vi "Read Display Name.vi"(11 "Assert Display in":refnum<class "Assert Display.lvclass">) -> (2 "Display Name":string)   [LabVIEW 2016, in "Assert API Components.lvlib" / "Assert Display.lvlib" / "Assert Display.lvclass"]
uses:
  Assert Display.lvclass
  Assert Display.lvclass/Assert Display.ctl
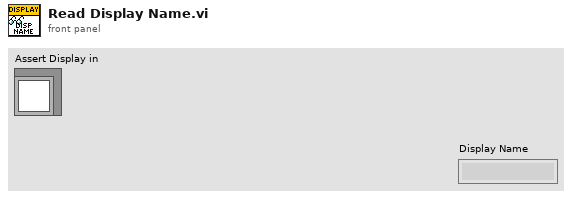
[diagram p1: front panel]
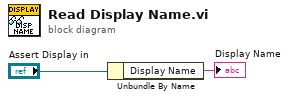
[diagram p0: block diagram]
diagram:
  n1 = Unbundle By Name("Assert Display in") -> ("Display Name"=→"Display Name":string)
